vi "ReleaseSemaphore.vi"(0 "reference in":refnum<class "VdTcpIP.lvclass">, 2 "ManagedToLockIt":bool, 5 "error in (no error)":errorcluster) -> (14 "reference out":refnum<class "VdTcpIP.lvclass">, 19 "error out":errorcluster)   [LabVIEW 2020, in "VdTcpIP.lvclass"]
uses:
  VdTcpIP.lvclass
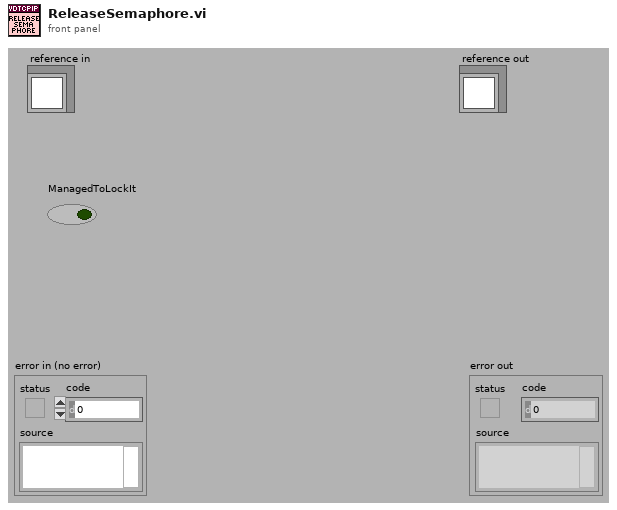
[diagram p1: front panel]
types:
  T1 = typedef "VdTcpIP.lvclass/ObjectAttributes.ctl" = cluster{"IP-Address":string, "Port":u16, "Connection":refnum<k5>, "Listener":refnum<k5>, "ListenerConnection":refnum<k5>, "Listner":bool, "ListnerProcessRunning":bool, "InConnections":refnum<k5>[], "InConnectionsIP":string[], "InConnectionAdded":refnum<notifier>, "RunVIOnNewConnection":variant, "DataToNewConnectionVI":cluster{"ControlName":string, "ControlValue":variant}[], "WebServicesURL_Location(http://...)":string, "WebServicesPostWebPage(*.asmx)":string, "Semaphore":T2, "AutoReConnectTimes":i32, "AutoReConnectInterval(ms)":i32, "ConnectionTimeout":i32}
  T2 = typedef "Semaphore RefNum" = refnum<k1>
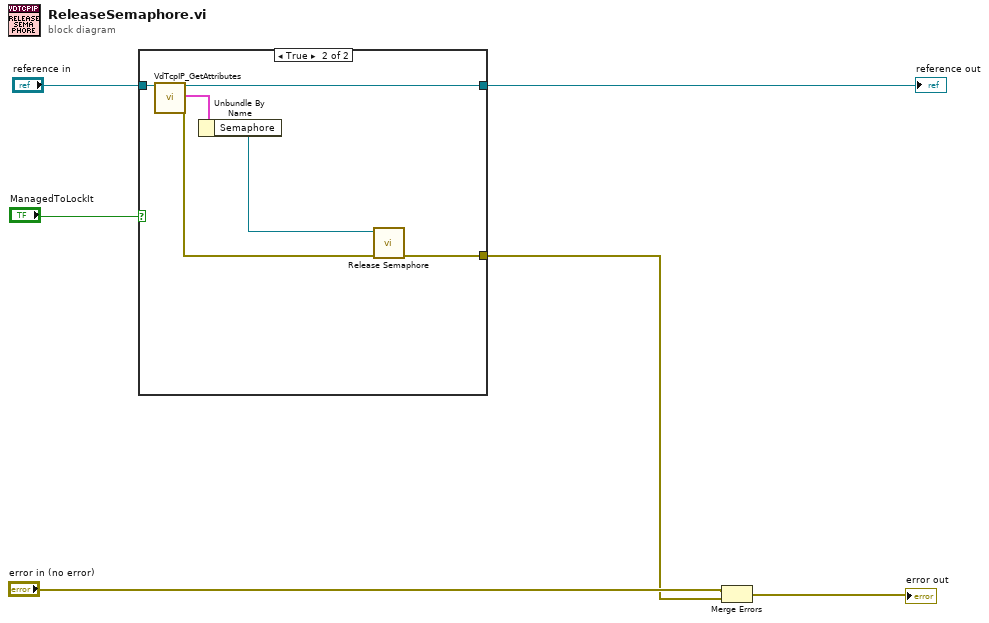
[diagram p0: block diagram]
diagram:
  n1 = case shown="True" "ManagedToLockIt" {
    tunnel: "reference in" -> [w7 w13]
    tunnel: [w7 w12] -> w5
    tunnel: [_ w9] -> w3
    frame False {
    }
    frame True {
      n2 = call "VdTcpIP_GetAttributes.vi"("reference in"=w13) -> ("reference out"=w12:refnum<class "VdTcpIP.lvclass">, "Data"=w8:T1, "error out"=w10:errorcluster)  [unwired: 15 in, 1 out]
      n3 = Unbundle By Name(w8) -> ("Semaphore"=w11:T2)
      n4 = call <vilib>:"Release Semaphore.vi"("error in (no error)"=w10, "semaphore"=w11) -> ("error out"=w9:errorcluster)  [unwired: 4 in, 1 out]
    }
  }
  "reference out" <- w5
  n5 = Merge Errors("error in (no error)", w3) -> (→"error out":errorcluster)
